vi "estimateSize.vi"(8 "error in (no error)":errorcluster, 10 "imageArray":dbl[][](array[numeric]), 11 "BECImageProcessor in":refnum<class "BECImageProcessor.lvclass">) -> (0 "error out":errorcluster, 1 "y Dimension":i32, 2 "x Dimension":i32, 3 "BECImageProcessor out":refnum<class "BECImageProcessor.lvclass">)   [LabVIEW 2011, in "Tools.lvlib" / "Imaging.lvlib" / "BECImageProcessor.lvclass"]
uses:
  BECImageProcessor.lvclass
panel:
  in  "Path":path
  out "integralNumeric":dbl
  out "Image":T1(plugin-control)
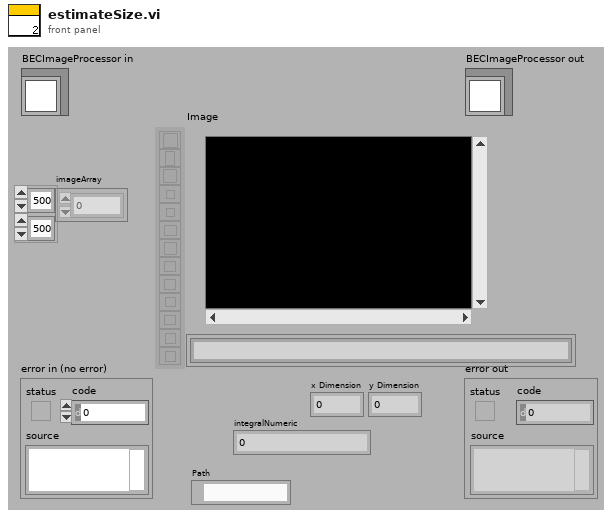
[diagram p1: front panel]
types:
  T1 = typedef "IMAQ Image.ctl" = refnum<image>
  T2 = cluster{"Objects":u16, "Threshold":i32, "Reject Border":bool, "Fill Holes":bool, "Min Object Size":bool, "Min Size":i32, "Max Object Size":bool, "Max Size":i32, "Show Search Area":bool, "Show Center":bool, "Show Bounding Box":bool}
  T3 = typedef "Image Type" = u32
  T4 = cluster{"Object Center":cluster{"X":sgl, "Y":sgl}, "Bounding Box":cluster{"X Left":i32, "Y Top":i32, "X Right":i32, "Y Bottom":i32}, "Area":sgl, "Orientation":sgl, "Aspect Ratio":sgl, "Nb Holes":i32}[]
  T5 = cluster{"Object Center":cluster{"X":sgl, "Y":sgl}, "Bounding Box":cluster{"X Left":i32, "Y Top":i32, "X Right":i32, "Y Bottom":i32}, "Area":sgl, "Orientation":sgl, "Aspect Ratio":sgl, "Nb Holes":i32}
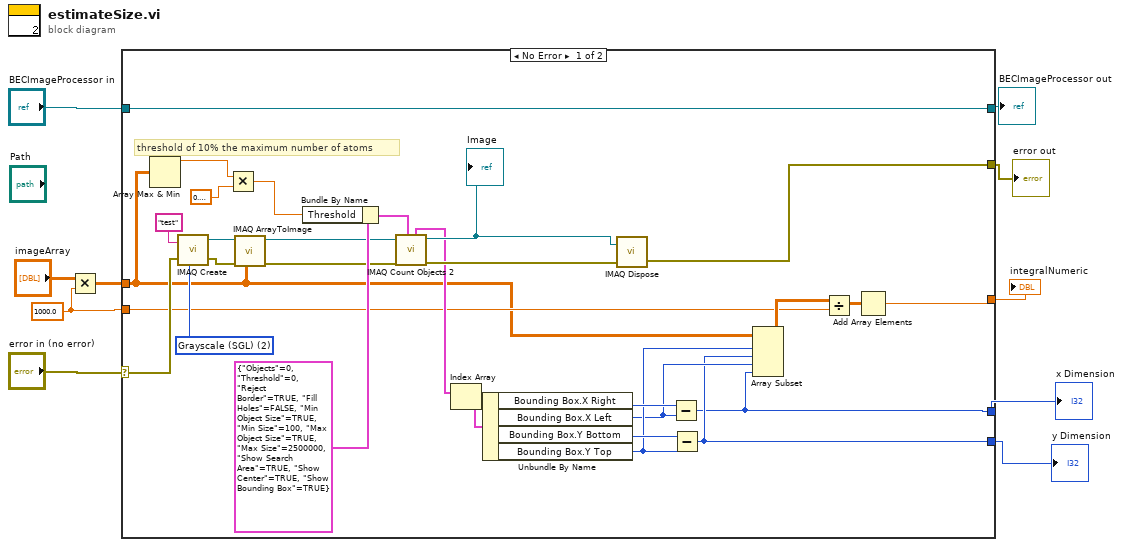
[diagram p0: block diagram]
diagram:
  w1 = 1000.0
  n1 = Multiply(x="imageArray", y=w1) -> (x*y=w2:dbl[][])
  n2 = case shown="No Error" "error in (no error)" {
    selector: "error in (no error)" -> [w37 w41]
    tunnel: [w33 w41] -> w9
    tunnel: [w39 w40] -> w7
    tunnel: "BECImageProcessor in" -> [w39 w40]
    tunnel: [w21 _] -> w6
    tunnel: [w22 _] -> w5
    tunnel: [w17 _] -> w4
    tunnel: w2 -> [w11 _]
    tunnel: w1 -> [w16 _]
    frame No Error {
      w36 = T3 2 items=["Grayscale (U8)", "Grayscale (I16)", "Grayscale (SGL)", "Complex (CSG)", "RGB (U32)", "HSL (U32)", "RGB (U64)"] ("Image Type")
      # "threshold of 10% the maximum number of atoms"
      n3 = Array Max & Min(array=w11) -> (max value=w30:dbl)  [unwired: 3 out]
      n4 = call "IMAQ Create"("Image Name"="test", "Image Type"=w36, "error in (no error)"=w37) -> ("New Image"=w15:T1, "error out"=w14:errorcluster)  [unwired: 2 in]
      n5 = Multiply(x=w30, y=0.36787944117144233) -> (x*y=w27:dbl)
      n6 = call "IMAQ ArrayToImage"("Image Pixels (Float)"=w11, "error in (no error)"=w14, "Image"=w15) -> ("error out"=w13:errorcluster, "Image Out"=w12:T1)  [unwired: 7 in]
      n7 = Bundle By Name(cluster=T2 {"Objects"=0, "Threshold"=0, "Reject Border"=TRUE, "Fill Holes"=FALSE, "Min Object Size"=TRUE, "Min Size"=100, "Max Object Size"=TRUE, "Max Size"=2500000, "Show Search Area"=TRUE, "Show Center"=TRUE, "Show Bounding Box"=TRUE} ("Settings"), "Threshold"=w27) -> (w28:T2)
      n8 = call "IMAQ Count Objects 2"("Settings"=w28, "error in (no error)"=w13, "Image"=w12) -> ("error out"=w34:errorcluster, "Image Out"=w35:T1, "Objects"=w32:T4)  [unwired: 4 in, 2 out]
      "Image" <- w35
      n9 = Index Array(array=w32) -> (element=w31:T5)  [unwired: 1 in]
      n10 = Unbundle By Name(w31) -> ("Bounding Box.X Right"=w26:i32, "Bounding Box.X Left"=w23:i32, "Bounding Box.Y Bottom"=w25:i32, "Bounding Box.Y Top"=w24:i32)
      n11 = call "IMAQ Dispose"("Image"=w35, "error in (no error)"=w34) -> ("error out"=w33:errorcluster)  [unwired: 4 in]
      n12 = Subtract(x=w26, y=w23) -> (x-y=w21:i32)
      n13 = Subtract(x=w25, y=w24) -> (x-y=w22:i32)
      n14 = Array Subset(array=w11, index (row)=w24, length (row)=w22, index (col)=w23, length (col)=w21) -> (w20:dbl[][])
      n15 = Divide(x=w20, y=w16) -> (x/y=w19:dbl[][])
      n16 = Add Array Elements(numeric array=w19) -> (sum=w17:dbl)
    }
    frame Error {
    }
  }
  "error out" <- w9
  "BECImageProcessor out" <- w7
  "x Dimension" <- w6
  "y Dimension" <- w5
  "integralNumeric" <- w4
